vi "Stop Core.vi"(10 "final error code":i32, 11 "LoggingActor in":refnum<class "LoggingActor.lvclass">) -> (3 "LoggingActor out":refnum<class "LoggingActor.lvclass">)   [LabVIEW 2022 SP3, in "LoggingActor.lvlib" / "LoggingActor.lvclass"]
doc: "(<B>Filename</B>: Actor Framework.lvlib:Actor.lvclass:Stop Core.vi)\n\nDefines what the actor does before it stops. Use the <B>final error code</B> input to determine whether the actor shut down in response to an error.\n\nBy default, this method does nothing. A descendant class may override it to define behavior, such as shutting down any processes the actor initiated in its override of the Actor Core method."
uses:
  LoggingActor.lvclass
  LoggingActor.lvclass/LoggingActor.ctl
  <vilib>/ActorFramework/Actor/Actor.lvclass
  Logger/Source/Logger/Logger.lvclass
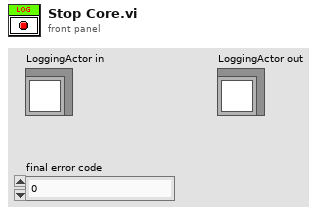
[diagram p1: front panel]
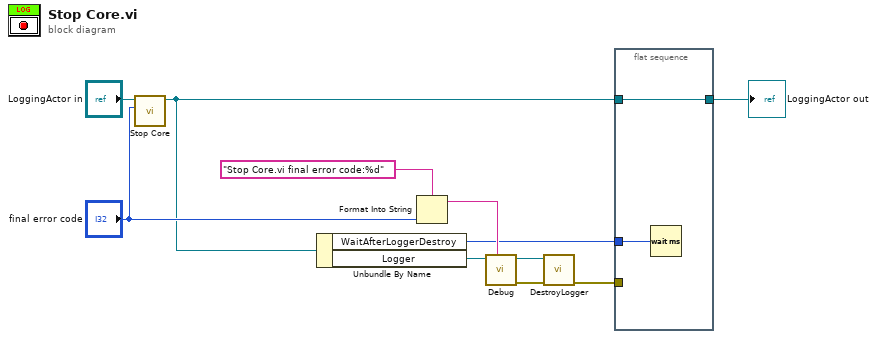
[diagram p0: block diagram]
diagram:
  n1 = call-parent "Stop Core.vi"("final error code"="final error code", "Actor in"="LoggingActor in") -> ("Actor out"=w2:refnum<class "LoggingActor.lvclass">)  [unwired: 9 in]
  n2 = Unbundle By Name(w2) -> ("WaitAfterLoggerDestroy"=w1:u32, "Logger"=w10:refnum<class "Logger.lvclass">)
  n3 = Format Into String(format string="Stop Core.vi final error code:%d" ("Message"), "final error code") -> (resulting string=w8:string)  [unwired: 2 in, 1 out]
  n4 = call-dynamic "Debug.vi"("Message"=w8, "Logger in"=w10) -> ("error out"=w4:errorcluster, "Logger out"=w9:refnum<class "Logger.lvclass">)  [unwired: 8 in]
  n5 = call-dynamic "DestroyLogger.vi"("error in (no error)"=w4, "Logger in"=w9) -> ("error out"=w5:errorcluster)  [unwired: 9 in]
  n6 = flat-sequence {
    tunnel: w5 -> [_]
    tunnel: [w13] -> w3
    tunnel: w2 -> [w13]
    tunnel: w1 -> [w12]
    frame #0 {
      n7 = Wait (ms)(milliseconds to wait=w12) -> ()  [unwired: 1 out]
    }
  }
  "LoggingActor out" <- w3
